vi "Read Path Commands.vi"(8 "error in (no error)":errorcluster, 11 "Path in":refnum<class "Path.lvclass">) -> (0 "error out":errorcluster, 2 "Path Commands":refnum<class "PathCommands.lvclass">[](array[class]), 3 "Path out":refnum<class "Path.lvclass">)   [LabVIEW 2019, in "Path.lvclass"]
uses:
  Path.lvclass
  PathCommands/PathCommands.lvclass
  Path.lvclass/Path.ctl
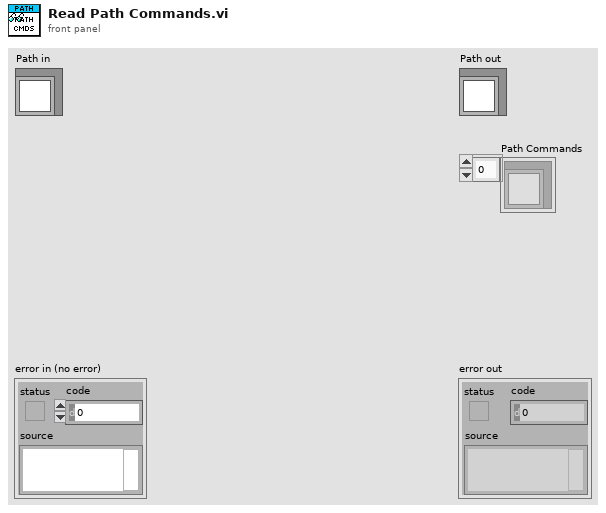
[diagram p1: front panel]
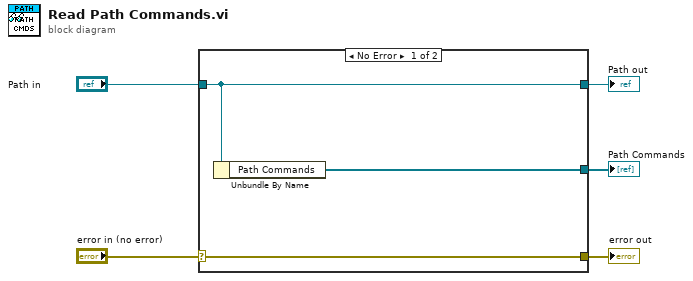
[diagram p0: block diagram]
diagram:
  n1 = case shown="No Error" "error in (no error)" {
    selector: "error in (no error)" -> [w8 w9]
    tunnel: [w8 w9] -> w4
    tunnel: [w6 w10] -> w2
    tunnel: "Path in" -> [w6 w10]
    tunnel: [w7 _] -> w1
    frame No Error {
      n2 = Unbundle By Name(w6) -> ("Path Commands"=w7:refnum<class "PathCommands.lvclass">[])
    }
    frame Error {
    }
  }
  "error out" <- w4
  "Path out" <- w2
  "Path Commands" <- w1
